vi "AnalyseViIcon.vi"(1 "ViRef":refnum<vi>, 5 "error in (no error)":errorcluster) -> (10 "FrameColor":u32(colorbox), 12 "FrameThickness(1)":u32=1, 13 "ValidIcon":bool, 15 "HeaderIcon":u8[][](array[numeric]) format="%x", 16 "HeaderBkColor":u32(colorbox), 17 "BodyIcon":u8[][](array[numeric]) format="%x", 18 "BodyBkColor":u32(colorbox), 19 "error out":errorcluster)   [LabVIEW 2010]
uses:
  <vilib>/Analysis/NI_AALBase.lvlib
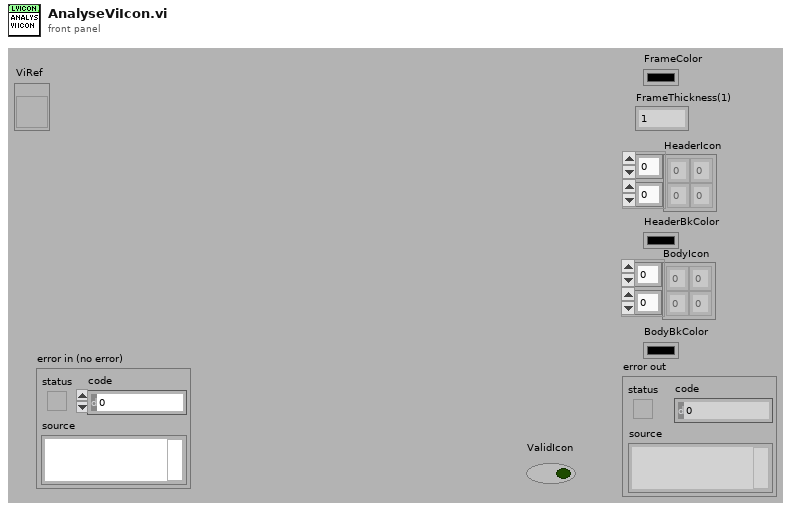
[diagram p1: front panel]
types:
  T1 = cluster{"image":u8[][], "FrameThickness":i32, "FrameColor":u32, "HeaderBkColor":u32, "BodyBkColor":u32, "SplitterAtRow":i32, "Header":u8[][], "Body":u8[][]}
  T2 = typedef "imagedata.ctl" = cluster{"image type":i32, "image depth":i32, "image":u8[], "mask":u8[], "colors":u32[], "Rectangle":cluster{"left":i16, "top":i16, "right":i16, "bottom":i16}}
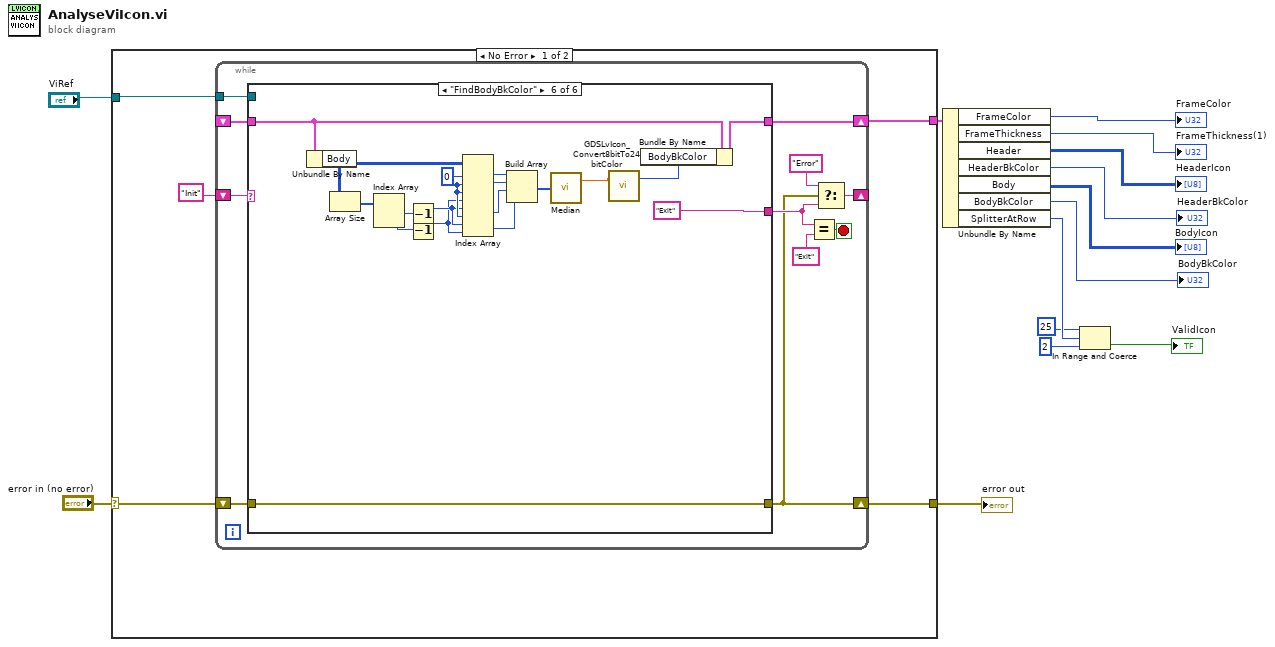
[diagram p0: block diagram]
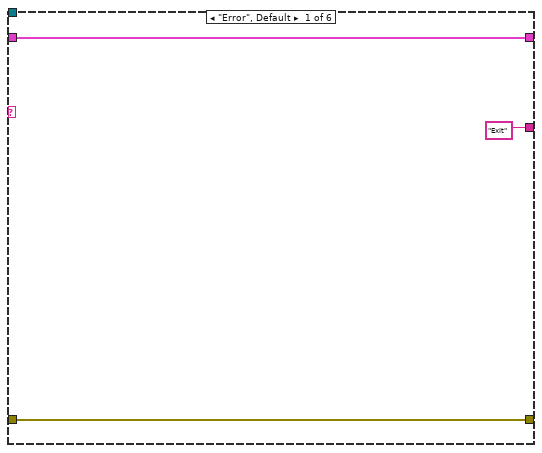
[diagram p2: hidden frame]
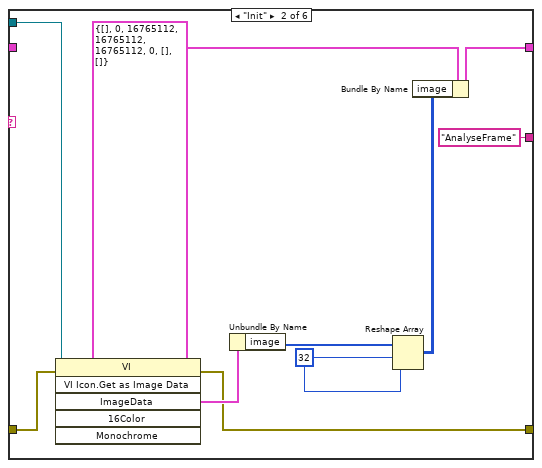
[diagram p3: hidden frame]
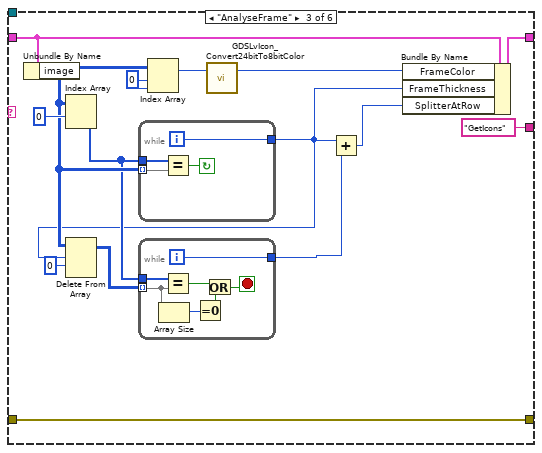
[diagram p4: hidden frame]
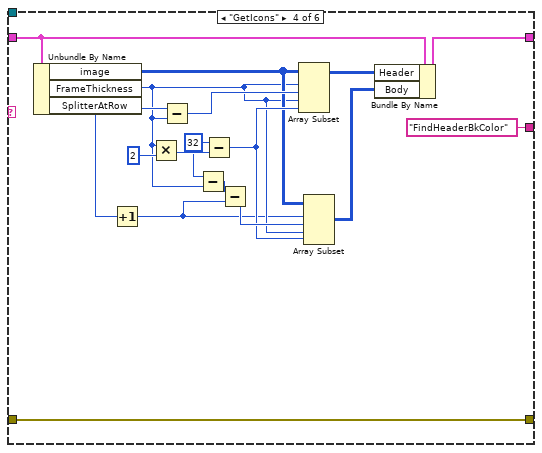
[diagram p5: hidden frame]
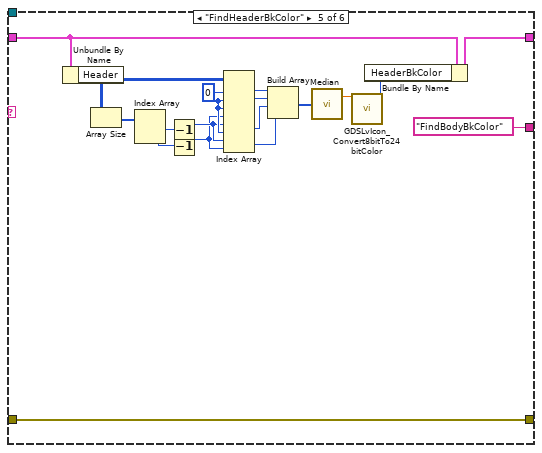
[diagram p6: hidden frame]
diagram:
  n1 = case shown="No Error" "error in (no error)" {
    selector: "error in (no error)" -> [w18 w123]
    tunnel: "ViRef" -> [w16 _]
    tunnel: [w17 w123] -> w13
    tunnel: [w15 _] -> w12
    frame No Error {
      n2 = while {
        shift-right: [w23] -> w17
        shift-left: w18 -> [w30]
        shift-right: [w28] -> _
        shift-left: "Init" -> [w29]
        shift-right: [w22] -> w15
        shift-left: _ -> [w21]
        tunnel: w16 -> [w20]
        stop <- w27 stop-if-true
        n3 = case shown="\"FindBodyBkColor\"" w29 {
          tunnel: w30 -> [w33 w42 w46 w79 w103 w121]
          tunnel: [w33 w34 w46 w79 w103 w121] -> w23
          tunnel: ["Exit" "AnalyseFrame" "GetIcons" "FindHeaderBkColor" "FindBodyBkColor" "Exit"] -> w24
          tunnel: [w31 w37 w56 w85 w101 w119] -> w22
          tunnel: w21 -> [w31 _ w57 w86 w102 w120]
          tunnel: w20 -> [_ w35 _ _ _ _]
          frame "Error", Default {
          }
          frame "Init" {
            w39 = 32 ("dimension size")
            n4 = invoke class="VI" method="VI Icon.Get as Image Data"(reference=w35, error in=w42) -> (error out=w34:errorcluster, "ImageData"=w41:T2)  [unwired: 4 in, 4 out]
            n5 = Unbundle By Name(w41) -> ("image"=w40:u8[])
            n6 = Reshape Array(w40, w39, w39) -> (w36:u8[][])
            n7 = Bundle By Name(cluster=T1 {"image"=[], "FrameThickness"=0, "FrameColor"=16765112, "HeaderBkColor"=16765112, "BodyBkColor"=16765112, "SplitterAtRow"=0, "Header"=[], "Body"=[]}, "image"=w36) -> (w37:T1)
          }
          frame "AnalyseFrame" {
            w55 = 0 ("index (row)")
            n8 = Unbundle By Name(w57) -> ("image"=w51:u8[][])
            n9 = Index Array(array=w51, index (row)=0) -> (element=w50:u8[])  [unwired: 1 in]
            n10 = while {
              tunnel: w51 -> [w69] mode=indexing
              tunnel: w50 -> [w68]
              tunnel: [w66] -> w45
              i -> [w66]
              stop <- w67 continue-if-true
              n11 = Equal?(x=w68, y=w69) -> (x = y?=w67:bool)
            }
            n12 = Delete From Array(array=w51, length=w45, index (row)=0) -> (array with subset deleted=w49:u8[][])  [unwired: 1 in, 1 out]
            n13 = while {
              tunnel: w49 -> [w62] mode=indexing
              tunnel: w50 -> [w65]
              tunnel: [w63] -> w44
              i -> [w63]
              stop <- w61 stop-if-true
              n14 = Array Size(array=w62) -> (size(s)=w60:i32)
              n15 = Equal?(x=w65, y=w62) -> (x = y?=w64:bool)
              n16 = Equal To 0?(x=w60) -> (x = 0?=w59:bool)
              n17 = Or(x=w64, y=w59) -> (x .or. y?=w61:bool)
            }
            n18 = Index Array(array=w51, index (row)=w55, index (col)=w55) -> (element=w54:u8)
            n19 = call "GDSLvIcon_Convert24bitTo8bitColor.vi"("Color 24bit In"=w54) -> ("Adjusted 24bit Color Out"=w53:u32)  [unwired: 15 in, 3 out]
            n20 = Add(x=w45, y=w44) -> (x+y=w47:i32)
            n21 = Bundle By Name(cluster=w57, "FrameColor"=w53, "FrameThickness"=w45, "SplitterAtRow"=w47) -> (w56:T1)
          }
          frame "GetIcons" {
            w73 = 32 ("x")
            n22 = Unbundle By Name(w86) -> ("image"=w74:u8[][], "FrameThickness"=w72:i32, "SplitterAtRow"=w78:i32)
            n23 = Increment(x=w78) -> (x+1=w70:i32)
            n24 = Multiply(x=w72, y=2) -> (x*y=w80:i32)
            n25 = Subtract(x=w78, y=w72) -> (x-y=w82:i32)
            n26 = Subtract(x=w73, y=w72) -> (x-y=w71:i32)
            n27 = Subtract(x=w73, y=w80) -> (x-y=w76:i32)
            n28 = Subtract(x=w71, y=w70) -> (x-y=w77:i32)
            n29 = Array Subset(array=w74, index (row)=w72, length (row)=w82, index (col)=w72, length (col)=w76) -> (w83:u8[][])
            n30 = Array Subset(array=w74, index (row)=w70, length (row)=w77, index (col)=w72, length (col)=w76) -> (w75:u8[][])
            n31 = Bundle By Name(cluster=w86, "Header"=w83, "Body"=w75) -> (w85:T1)
          }
          frame "FindHeaderBkColor" {
            w96 = 0 ("index (row)")
            n32 = Unbundle By Name(w102) -> ("Header"=w99:u8[][])
            n33 = Array Size(array=w99) -> (size(s)=w100:i32[])
            n34 = Index Array(array=w100) -> (element #1=w98:i32, element #2=w97:i32)  [unwired: 2 in]
            n35 = Decrement(x=w98) -> (x-1=w95:i32)
            n36 = Decrement(x=w97) -> (x-1=w94:i32)
            n37 = Index Array(array=w99, index (row) #1=w96, index (col) #1=w96, index (row) #2=w96, index (col) #2=w94, index (row) #3=w95, index (col) #3=w96, index (row) #4=w95, index (col) #4=w94) -> (element #1=w93:u8, element #2=w92:u8, element #3=w91:u8, element #4=w90:u8)
            n38 = Build Array(w93, w92, w91, w90) -> (w89:u8[])
            n39 = call <vilib>:"Median.vi"("X"=w89) -> ("median"=w88:dbl)  [unwired: 1 out]
            n40 = call "GDSLvIcon_Convert8bitTo24bitColor.vi"("Color8bit"=w88) -> ("Color24bit"=w87:u32)  [unwired: 17 in, 1 out]
            n41 = Bundle By Name(cluster=w102, "HeaderBkColor"=w87) -> (w101:T1)
          }
          frame "FindBodyBkColor" {
            w114 = 0 ("index (row)")
            n42 = Unbundle By Name(w120) -> ("Body"=w117:u8[][])
            n43 = Array Size(array=w117) -> (size(s)=w118:i32[])
            n44 = Index Array(array=w118) -> (element #1=w116:i32, element #2=w115:i32)  [unwired: 2 in]
            n45 = Decrement(x=w116) -> (x-1=w113:i32)
            n46 = Decrement(x=w115) -> (x-1=w112:i32)
            n47 = Index Array(array=w117, index (row) #1=w114, index (col) #1=w114, index (row) #2=w114, index (col) #2=w112, index (row) #3=w113, index (col) #3=w114, index (row) #4=w113, index (col) #4=w112) -> (element #1=w111:u8, element #2=w110:u8, element #3=w109:u8, element #4=w108:u8)
            n48 = Build Array(w111, w110, w109, w108) -> (w107:u8[])
            n49 = call <vilib>:"Median.vi"("X"=w107) -> ("median"=w106:dbl)  [unwired: 1 out]
            n50 = call "GDSLvIcon_Convert8bitTo24bitColor.vi"("Color8bit"=w106) -> ("Color24bit"=w105:u32)  [unwired: 17 in, 1 out]
            n51 = Bundle By Name(cluster=w120, "BodyBkColor"=w105) -> (w119:T1)
          }
        }
        n52 = Equal?(x=w24, y="Exit") -> (x = y?=w27:bool)
        n53 = Select(t="Error", s=w23, f=w24) -> (s? t:f=w28:string)
      }
    }
    frame Error {
    }
  }
  "error out" <- w13
  n54 = Unbundle By Name(w12) -> ("FrameColor"=→"FrameColor":u32, "FrameThickness"=→"FrameThickness(1)":i32, "Header"=→"HeaderIcon":u8[][], "HeaderBkColor"=→"HeaderBkColor":u32, "Body"=→"BodyIcon":u8[][], "BodyBkColor"=→"BodyBkColor":u32, "SplitterAtRow"=w4:i32)
  n55 = In Range and Coerce(upper limit=25 ("x"), x=w4, lower limit=2) -> (In Range?=→"ValidIcon":bool)  [unwired: 1 out]
